vi "实例37 三维曲面图.vi"() -> ()   [LabVIEW 2014]
uses:
  <vilib>/Platform/NI_3dgraph.lvlib
panel:
  in  "3D Surface":refnum<k7>(container) caption="三维曲面"
  # "三维图的显示"
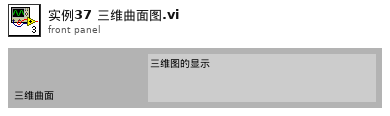
[diagram p1: front panel]
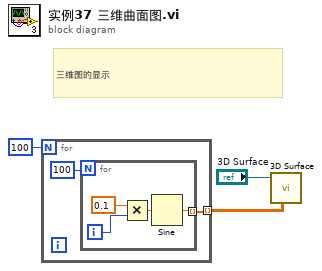
[diagram p0: block diagram]
diagram:
  # "三维图的显示"
  n1 = for {
    N: 100 -> [_]
    tunnel: [w4] -> w1 mode=indexing
    n2 = for {
      N: 100 -> [_]
      tunnel: [w6] -> w4 mode=indexing
      i -> [w7]
      n3 = Multiply(x=0.1, y=w7) -> (x*y=w8:dbl)
      n4 = Sine(x=w8) -> (sin(x)=w6:dbl)
    }
  }
  n5 = call <vilib>:"3D Surface.vi"("z matrix"=w1, "3D graph"="3D Surface") -> ()  [unwired: 8 in, 2 out]
